vi "DSC Alarm Event Example.vi"() -> ()   [LabVIEW 2021, in "Dynamic Shared Variables.lvlib"]
uses:
  Dynamic Shared Variables.lvlib
  Alarm Cluster (UI).ctl
  Alarm Cluster.ctl
  <vilib>/Utility/miscctls.llb/LVMouseTypeDef.ctl
  Tag VIs/Tag FGV Operation Enum.ctl
  Alarm Log Operation Enum.ctl
  <vilib>/lvdsc/NI_DSC.lvlib
  Waveform Loop/Waveform Loop.lvlib
panel:
  out "Alarm CSV Logfile path":path
  out "Alarm Event Time":timestamp
  in  "Tag Value":dbl=80.0 format="%#_13g"
  in  "Write Tag Value":bool
  in  "numeric alarm settings":T1={"enable? (F)"=TRUE, "name"="HiHi", "alarm type"=enum."HI_HI", "level/change"=50.0, "deadband/time"=1.0, "priority"=1, "ack type"=enum."Each Occurrence", "area"="", "description"="", "log? (T)"=TRUE}
  in  "Create Shared Variable":bool
  out "Alarm Model":T2[](array[typedef]) {"Alarm"."value" format="%.2f"; "Alarm"."setpoint" format="%.2f"; "Alarm"."clear time" format="%<%X\n%x>T"; "Alarm"."ack time" format="%<%X\n%x>T"; "Alarm"."set time" format="%<%X\n%x>T"}
  in  "Alarms":T3[](array[typedef])
  in  "stop":bool
  # "Instructions\n1. Press Create Shared Variable button with designated HI_HI threshold.\n2. Press Write Tag Value to write a Tag Value that is above the HI_HI threshold.\n3. Observe that the Alarm Event was triggered when the Alarm Event Time changes.\n4. Observer that the HIHi alarm is displayed in the alarm array."
  # "2."
  # "1."
  # "3."
  # "4."
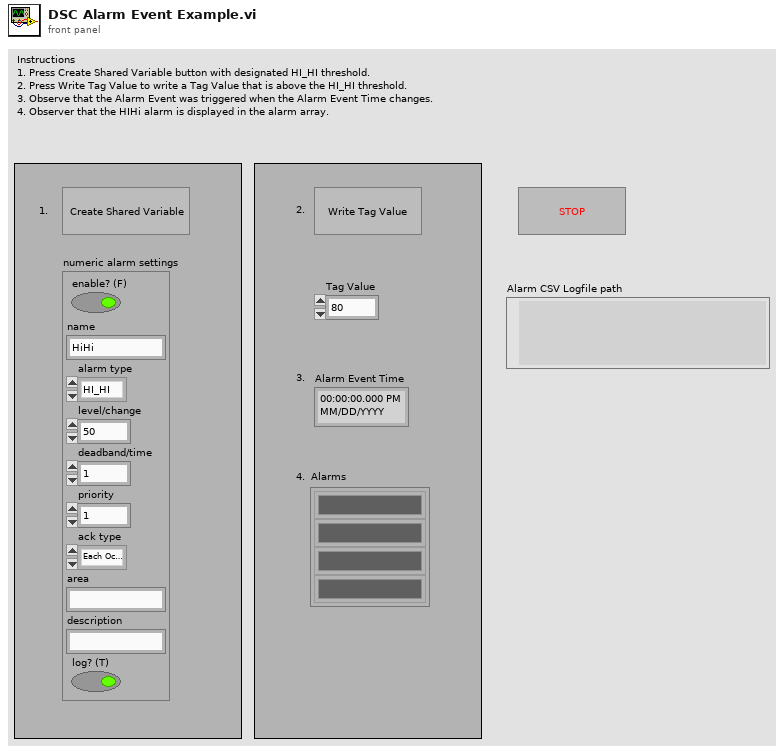
[diagram p1: front panel]
types:
  T1 = cluster{"enable? (F)":bool, "name":string, "alarm type":enum16{"HI_HI", "HI", "LO", "LO_LO"}, "level/change":dbl, "deadband/time":dbl, "priority":u32, "ack type":enum16{"Auto", "User", "None", "Each Occurrence"}, "area":string, "description":string, "log? (T)":bool}
  T2 = typedef "Dynamic Shared Variables.lvlib/Alarm Cluster.ctl" = cluster{"Color Box":u32, "Name":string, "Ack":bool, "Alarm":cluster{"alarm URL":string, "set time":timestamp, "set user":string, "ack time":timestamp, "ack user":string, "clear time":timestamp, "clear user":string, "setpoint":dbl, "value":dbl, "priority":u32, "alarm area":string, "alarm description":string, "ack comment":string, "event?":bool, "Refnum":u64}}
  T3 = typedef "Dynamic Shared Variables.lvlib/Alarm Cluster (UI).ctl" = cluster{"Color Box":u32, "Name":string, "Ack":bool}
  T4 = typedef "Alarm Log Operation Enum.ctl" = enum16{"Create Log", "Log Alarm", "Close Log"}
  T5 = typedef "Tag FGV Operation Enum.ctl" = enum16{"Init", "Set Notification Queue", "Create Tag", "Commit", "Write Tag (Numeric)", "Write Tag (Boolean)", "Read All Tags", "Read One Tag", "Delete Tag Category", "Set Alarm Parameters (Numeric)", "Set Alarm Parameters (Boolean)", "Enable All Alarms", "Disable All Alarms", "Delete All Tags", "Read Alarms", "Ack Alarm", "Read Alarm Parameters (Numeric)", "Read Alarm Parameters (Boolean)"}
  T6 = typedef "LVMouseTypeDef.ctl" = cluster{"Mouse Position":cluster{"X":i32, "Y":i32}, "Mouse Modifiers":cluster{"Button Down":bool, "Shift Mod":bool, "Menu Mod":bool, "Option Mod":bool}}
  T7 = cluster{"Down":bool, "Mouse":T6, "Drag":bool, "Canvas":bool}
  T8 = enum32{"u32BitField", "bool", "double", "string", "int8", "uint8", "int16", "uint16", "int32", "uint32", "int64", "uint64", "single", "double waveform", "int16 waveform", "array of boolean", "array of int8", "array of uint8", "array of int16", "array of uint16", "array of int32", "array of uint32", "array of int64", "array of uint64", "array of single", "array of double", "array of double waveform", "array of int16 waveform", "array of string", "variant", "timestamp", "fixed point", "custom"}
  T9 = cluster{"alarm URL":string, "set time":timestamp, "set user":string, "ack time":timestamp, "ack user":string, "clear time":timestamp, "clear user":string, "setpoint":dbl, "value":dbl, "priority":u32, "alarm area":string, "alarm description":string, "ack comment":string, "event?":bool, "Refnum":u64}[]
  T10 = cluster{"alarm URL":string, "set time":timestamp, "set user":string, "ack time":timestamp, "ack user":string, "clear time":timestamp, "clear user":string, "setpoint":dbl, "value":dbl, "priority":u32, "alarm area":string, "alarm description":string, "ack comment":string, "event?":bool, "Refnum":u64}
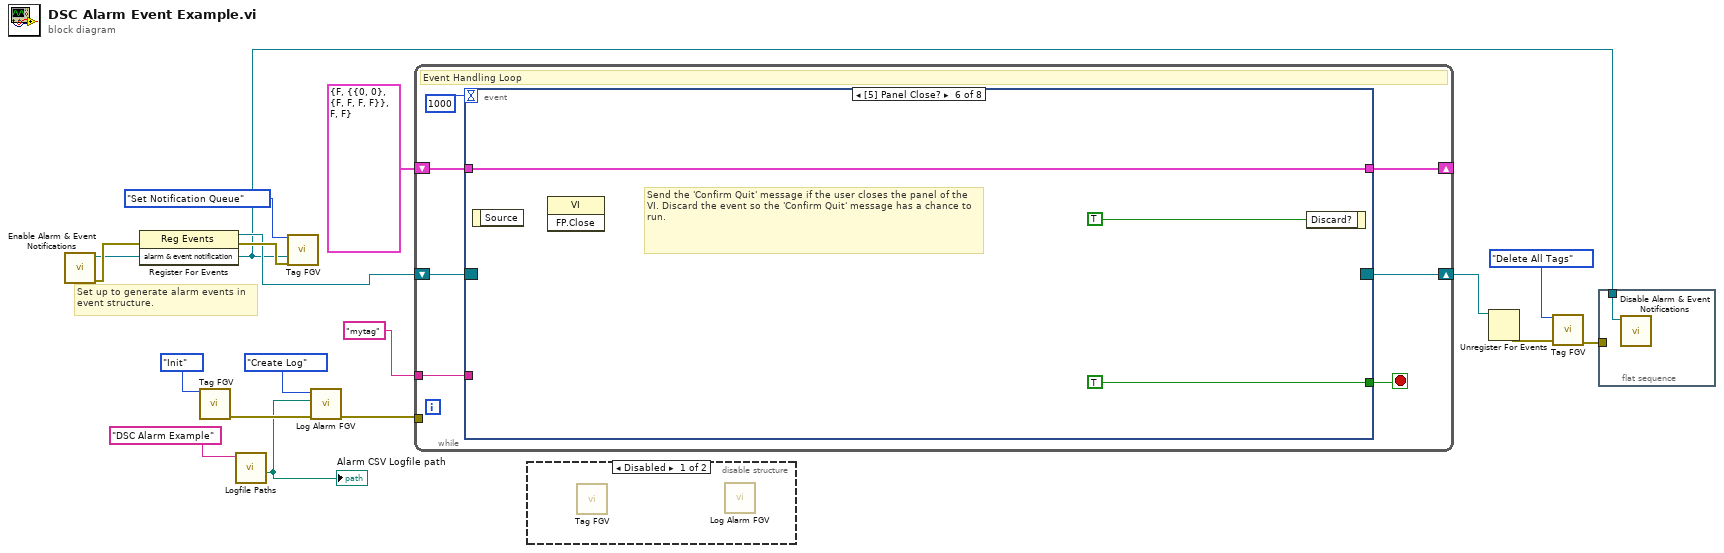
[diagram p0: block diagram]
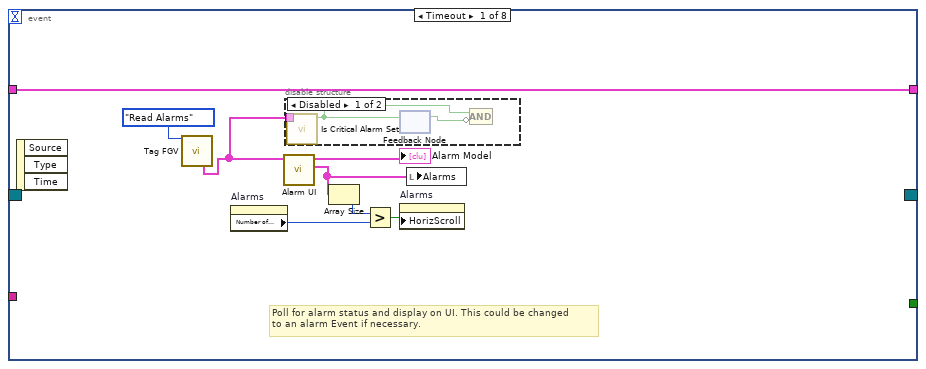
[diagram p3: hidden frame]
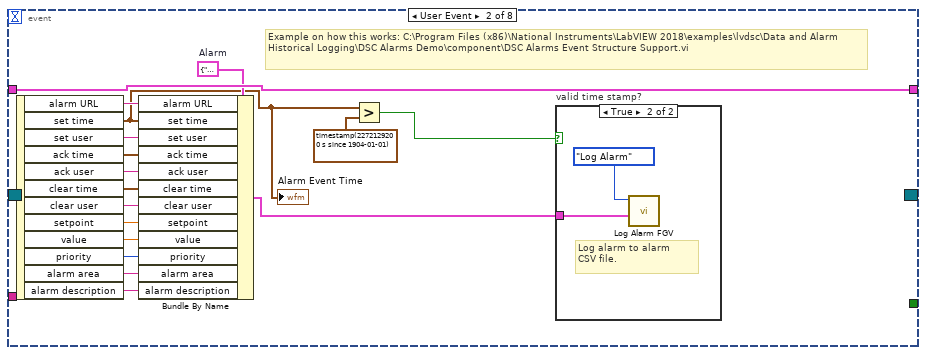
[diagram p5: hidden frame]
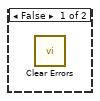
[diagram p6: hidden frame]
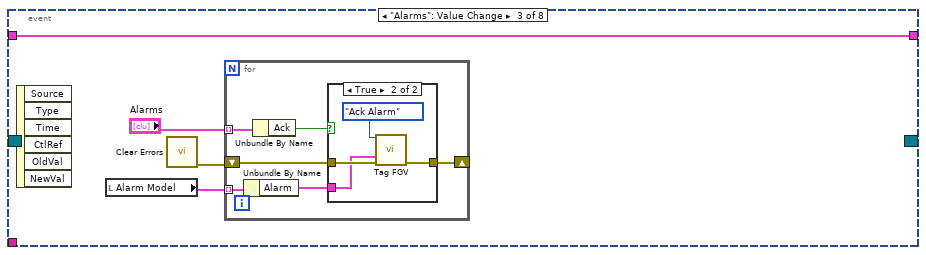
[diagram p7: hidden frame]
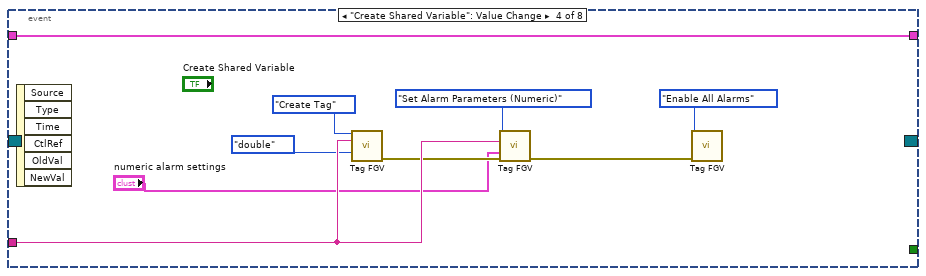
[diagram p9: hidden frame]
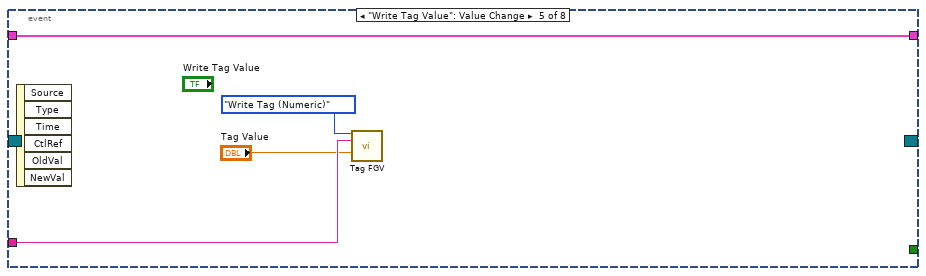
[diagram p10: hidden frame]
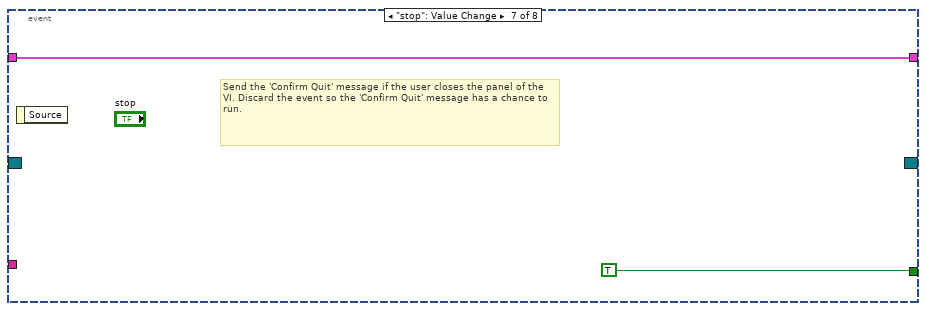
[diagram p11: hidden frame]
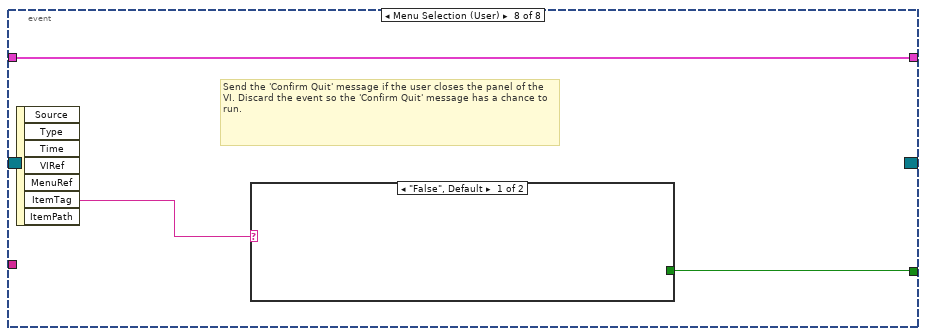
[diagram p12: hidden frame]
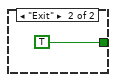
[diagram p13: hidden frame]
diagram:
  # "Set up to generate alarm events in\nevent structure."
  n1 = call <vilib>:"Enable Alarm & Event Notifications.vi"() -> ("error out"=w14:errorcluster, "alarm & event notification"=w2:refnum<user-event>)  [unwired: 10 in]
  n2 = register-events(error in=w14, w2) -> (reference out=w12:refnum<event-registration>, error out=w13:errorcluster)  [unwired: 1 in]
  n3 = call "Tag FGV.vi"("Operation"=Tag_FGV_Operation_Enum."Init") -> ("error out"=w6:errorcluster)  [unwired: 7 in, 7 out]
  n4 = call "Logfile Paths.vi"("File Name"="DSC Alarm Example") -> ("Alarm CSV Logfile path"=w3:path)  [unwired: 8 in, 2 out]
  "Alarm CSV Logfile path" <- w3
  n5 = call "Tag FGV.vi"("Operation"=Tag_FGV_Operation_Enum."Set Notification Queue", "Data"=w2, "error in (no error)"=w13) -> ()  [unwired: 5 in, 8 out]
  n6 = call "Log Alarm FGV.vi"("error in (no error)"=w6, "Path"=w3, "Operation"=Alarm_Log_Operation_Enum."Create Log") -> ("error out"=w5:errorcluster)  [unwired: 8 in]
  n7 = while {
    shift-right: [w22] -> w17
    shift-left: w12 -> [w24]
    shift-right: [w20] -> _
    shift-left: T7 {"Down"=FALSE, "Mouse"={"Mouse Position"={"X"=0, "Y"=0}, "Mouse Modifiers"={"Button Down"=FALSE, "Shift Mod"=FALSE, "Menu Mod"=FALSE, "Option Mod"=FALSE}}, "Drag"=FALSE, "Canvas"=FALSE} -> [w21]
    tunnel: "mytag" ("Tag Name") -> [w19]
    tunnel: w5 -> [_]
    stop <- w23 stop-if-true
    # "Event Handling Loop"
    n8 = event shown="[5] Panel Close?" {
      selector: w24 -> [_ _ _ _ _ _ _ _]
      dyn-events: [_ _ _ _ _ _ _ _] -> w22
      timeout: 1000 -> [_ _ _ _ _ _ _ _]
      tunnel: [_ _ _ _ _ TRUE TRUE w90] -> w23
      tunnel: w21 -> [w32 w52 w55 w78 w82 w83 w86 w89]
      tunnel: [w32 w52 w55 w78 w82 w83 w86 w89] -> w20
      tunnel: w19 -> [_ _ _ w75 w80 _ _ _]
      event Timeout {
        # "Poll for alarm status and display on UI. This could be changed\nto an alarm Event if necessary."
        n9 = event-data() -> ()  [unwired: 1 in, 3 out]
        n10 = call "Tag FGV.vi"("Operation"=Tag_FGV_Operation_Enum."Read Alarms") -> ("alarms"=w26:T9)  [unwired: 7 in, 7 out]
        n11 = property on="Alarms" class="Arr (strict)"() -> ("Number of Columns"=w29:u32)  [unwired: 2 in, 2 out]
        n12 = call "Alarm UI.vi"("alarms"=w26) -> ("UI Alarms"=w31:T3[], "Alarm Model"=→"Alarm Model":T2[])  [unwired: 9 in]
        n13 = disable-structure shown="Disabled" {
          disable-tunnel: w26 -> [w35 _]
          frame Disabled {
            n14 = call "Is Critical Alarm Set.vi"("alarms"=w35) -> ("critical alarm?"=w33:bool)  [unwired: 10 in]
            n15 = feedback #1() -> (w34:bool)  [unwired: 1 in]
            n16 = feedback-in #1(w33) -> ()
            n17 = Compound Arithmetic op=AND(w33, invert w34) -> ()  [unwired: 1 out]
          }
          frame Enabled {
          }
        }
        n18 = Array Size(array=w31) -> (size(s)=w30:i32)
        n19 = Greater?(x=w30, y=w29) -> (0:w28:bool)
        n20 = property on="Alarms" class="Arr (strict)"("HorizScroll"=w28) -> ()  [unwired: 2 in, 2 out]
        n21 = local write "Alarms"(w31) -> ()
      }
      event User Event {
        w50 = T10 {"alarm URL"="", "set time"=timestamp(0 s since 1904-01-01), "set user"="", "ack time"=timestamp(0 s since 1904-01-01), "ack user"="", "clear time"=timestamp(0 s since 1904-01-01), "clear user"="", "setpoint"=0.0, "value"=0.0, "priority"=0, "alarm area"="", "alarm description"="", "ack comment"="", "event?"=FALSE, "Refnum"=0}  # Alarm
        # "Example on how this works: C:\\Program Files (x86)\\National Instruments\\LabVIEW 2018\\examples\\lvdsc\\Data and Alarm Historical Logging\\DSC Alarms Demo\\component\\DSC Alarms Event Structure Support.vi"
        n22 = event-data() -> ("alarm URL"=w49:string, "set time"=w48:timestamp, "set user"=w47:string, "ack time"=w46:timestamp, "ack user"=w45:string, "clear time"=w44:timestamp, "clear user"=w43:string, "setpoint"=w42:dbl, "value"=w41:dbl, "priority"=w38:u32, "alarm area"=w40:string, "alarm description"=w39:string)  [unwired: 1 in]
        "Alarm Event Time" <- w48
        n23 = Bundle By Name(cluster=w50, "alarm URL"=w49, "set time"=w48, "set user"=w47, "ack time"=w46, "ack user"=w45, "clear time"=w44, "clear user"=w43, "setpoint"=w42, "value"=w41, "priority"=w38, "alarm area"=w40, "alarm description"=w39) -> (w37:T10)
        n24 = Greater?(x=w48, y=timestamp(2272129200 s since 1904-01-01)) -> (0:w36:bool)
        n25 = case "valid time stamp?" shown="True" w36 {
          tunnel: w37 -> [_ w54]
          frame False {
            n26 = call <vilib>:"Clear Errors.vi"() -> ()  [unwired: 6 in, 2 out]
          }
          frame True {
            # "Log alarm to alarm\nCSV file."
            n27 = call "Log Alarm FGV.vi"("Alarm"=w54, "Operation"=Alarm_Log_Operation_Enum."Log Alarm") -> ()  [unwired: 9 in, 1 out]
          }
        }
      }
      event "Alarms": Value Change {
        n28 = event-data() -> ()  [unwired: 1 in, 6 out]
        n29 = local read "Alarm Model"() -> (w57:T2[])
        n30 = call <vilib>:"Clear Errors.vi"() -> ("error out"=w56:errorcluster)  [unwired: 6 in, 1 out]
        n31 = for {
          shift-right: [w63] -> _
          shift-left: w56 -> [w64]
          tunnel: "Alarms" -> [w62] mode=indexing
          tunnel: w57 -> [w60] mode=indexing
          n32 = Unbundle By Name(w60) -> ("Alarm"=w59:T10)
          n33 = Unbundle By Name(w62) -> ("Ack"=w61:bool)
          n34 = case shown="True" w61 {
            tunnel: w64 -> [w65 w69]
            tunnel: [w65 w68] -> w63
            tunnel: w59 -> [_ w66]
            frame False {
            }
            frame True {
              n35 = call "Tag FGV.vi"("Operation"=Tag_FGV_Operation_Enum."Ack Alarm", "Data"=w66, "error in (no error)"=w69) -> ("error out"=w68:errorcluster)  [unwired: 5 in, 7 out]
            }
          }
        }
      }
      event "Create Shared Variable": Value Change {
        n36 = event-data() -> ()  [unwired: 1 in, 6 out]
        n37 = call "Tag FGV.vi"("Operation"=Tag_FGV_Operation_Enum."Create Tag", "Tag Name"=w75, "Data"=T8."double" ("data type")) -> ("error out"=w74:errorcluster)  [unwired: 5 in, 7 out]
        n38 = call "Tag FGV.vi"("Operation"=Tag_FGV_Operation_Enum."Set Alarm Parameters (Numeric)", "Tag Name"=w75, "Data"="numeric alarm settings", "error in (no error)"=w74) -> ("error out"=w71:errorcluster)  [unwired: 4 in, 7 out]
        n39 = call "Tag FGV.vi"("Operation"=Tag_FGV_Operation_Enum."Enable All Alarms", "error in (no error)"=w71) -> ()  [unwired: 6 in, 8 out]
      }
      event "Write Tag Value": Value Change {
        n40 = event-data() -> ()  [unwired: 1 in, 6 out]
        n41 = call "Tag FGV.vi"("Operation"=Tag_FGV_Operation_Enum."Write Tag (Numeric)", "Tag Name"=w80, "Data"="Tag Value") -> ()  [unwired: 5 in, 8 out]
      }
      event Panel Close? {
        # "Send the 'Confirm Quit' message if the user closes the panel of the VI. Discard the event so the 'Confirm Quit' message has a chance to run."
        n42 = event-data() -> ()  [unwired: 1 in, 1 out]
        n43 = invoke class="VI" method="FP.Close"() -> ()  [unwired: 3 in, 3 out]
        n44 = event-data("Discard?"=TRUE) -> ()  [unwired: 1 in, 1 out]
      }
      event "stop": Value Change {
        # "Send the 'Confirm Quit' message if the user closes the panel of the VI. Discard the event so the 'Confirm Quit' message has a chance to run."
        n45 = event-data() -> ()  [unwired: 1 in, 1 out]
      }
      event Menu Selection (User) {
        # "Send the 'Confirm Quit' message if the user closes the panel of the VI. Discard the event so the 'Confirm Quit' message has a chance to run."
        n46 = event-data() -> ("ItemTag"=w88:string)  [unwired: 1 in, 6 out]
        n47 = case shown="\"False\", Default" w88 {
          tunnel: [_ TRUE] -> w90
          frame "False", Default {
          }
          frame "Exit" {
          }
        }
      }
    }
  }
  n48 = disable-structure shown="Disabled" {
    frame Disabled {
      n49 = call "Tag FGV.vi"() -> ()  [unwired: 8 in, 8 out]
      n50 = call "Log Alarm FGV.vi"() -> ()  [unwired: 11 in, 1 out]
    }
    frame Enabled {
    }
  }
  n51 = Unregister For Events(event registration refnum=w17) -> (error out=w8:errorcluster)  [unwired: 1 in]
  n52 = call "Tag FGV.vi"("Operation"=Tag_FGV_Operation_Enum."Delete All Tags", "error in (no error)"=w8) -> ("error out"=w1:errorcluster)  [unwired: 6 in, 7 out]
  n53 = flat-sequence {
    tunnel: w2 -> [w92]
    tunnel: w1 -> [_]
    frame #0 {
      n54 = call <vilib>:"Disable Alarm & Event Notifications.vi"("notification refnum"=w92) -> ()  [unwired: 10 in, 1 out]
    }
  }
